vi "DisplayBoard.vi"(11 "Board":refnum<class "Board.lvclass">) -> (3 "Array":u32[][](array[colorbox]))   [LabVIEW 2015, in "TronviewGame.lvlib"]
uses:
  TronviewGame.lvlib
  Board/Board.lvclass
  Board/Board.lvclass/Board.ctl
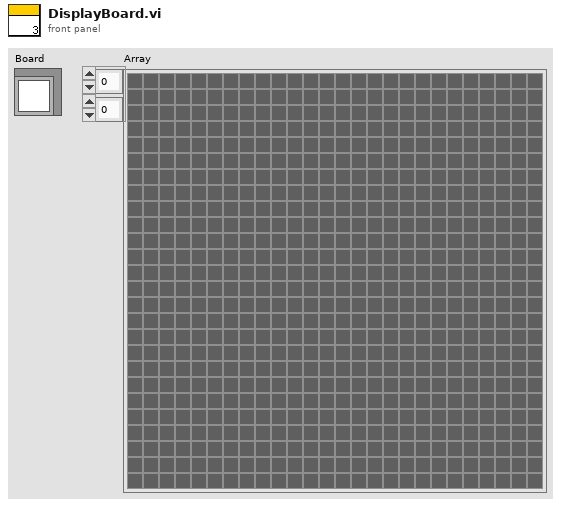
[diagram p1: front panel]
types:
  T1 = typedef "TronviewGame.lvlib/Board.lvclass/FieldState.ctl" = enum16{"Empty", "Blocked", "Player1Position", "Player2Postion", "Player1Marked", "Player2Marked"}
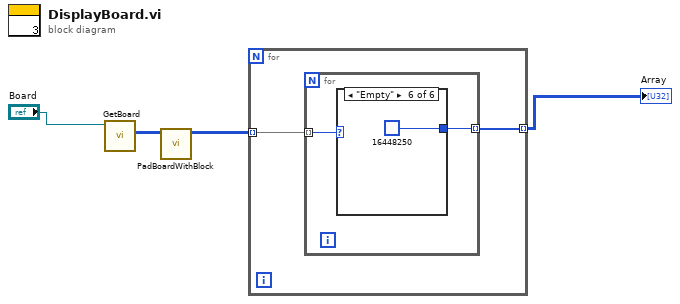
[diagram p0: block diagram]
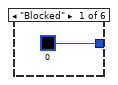
[diagram p2: hidden frame]
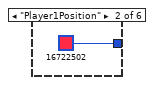
[diagram p3: hidden frame]
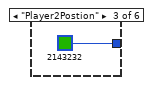
[diagram p4: hidden frame]
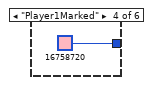
[diagram p5: hidden frame]
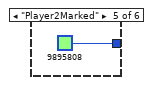
[diagram p6: hidden frame]
diagram:
  n1 = call "GetBoard.vi"("Board in"="Board") -> ("Board"=w2:T1[][])  [unwired: 8 in, 2 out]
  n2 = call "PadBoardWithBlock.vi"("Board"=w2) -> ("appended array"=w1:T1[][])  [unwired: 10 in]
  n3 = for {
    tunnel: w1 -> [w6] mode=indexing
    tunnel: [w5] -> w3 mode=indexing
    n4 = for {
      tunnel: w6 -> [w8] mode=indexing
      tunnel: [w7] -> w5 mode=indexing
      n5 = case shown="\"Empty\"" w8 {
        tunnel: [u32 0 u32 16722502 u32 2143232 u32 16758720 u32 9895808 u32 16448250] -> w7
        frame "Blocked" {
        }
        frame "Player1Position" {
        }
        frame "Player2Postion" {
        }
        frame "Player1Marked" {
        }
        frame "Player2Marked" {
        }
        frame "Empty" {
        }
      }
    }
  }
  "Array" <- w3
